vi "Configure Module.vi"   [LabVIEW 2020, in "NI ECAT Remote IO.lvlib"]
doc: "Configures a Remote I/O module."
uses:
  <vilib>/indcomecat/Remote IO/NI ECAT Remote IO.lvlib
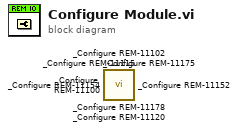
[diagram p0: block diagram]
diagram:
  n1 = call <vilib>:"_Configure REM-11178.vi"() -> ()  [unwired: 8 in, 4 out]
  n2 = call <vilib>:"_Configure REM-11175.vi"() -> ()  [unwired: 8 in, 4 out]
  n3 = call <vilib>:"_Configure REM-11154.vi"() -> ()  [unwired: 8 in, 4 out]
  n4 = call <vilib>:"_Configure REM-11152.vi"() -> ()  [unwired: 8 in, 4 out]
  n5 = call <vilib>:"_Configure REM-11120.vi"() -> ()  [unwired: 8 in, 4 out]
  n6 = call <vilib>:"_Configure REM-11102.vi"() -> ()  [unwired: 8 in, 4 out]
  n7 = call <vilib>:"_Configure REM-11115.vi"() -> ()  [unwired: 8 in, 4 out]
  n8 = call <vilib>:"_Configure REM-11100.vi"() -> ()  [unwired: 8 in, 4 out]
